vi "measure_max_power_stabilisation_keithley-2450.vi"(4 "Skip pixel?":bool, 5 "Date array":string[](array[string]), 6 "Scan settings":T1={"J-V scan"=TRUE, "Start voltage (V)"=0.0, "End voltage (V)"=0.0, "Step voltage (V)"=1.4, "Scan both directions"=TRUE, "Inverted device structure"=FALSE, "Settling delay (ms)"=10.0, "Measurement speed"=0, "Scan rate (V/s)"=0.0, "Stabilisation time (s)"=0.0, "Stabilisation mode"=0, "Stabilisation value (V or A) "=1.0, "Illumination"=0, "Stabilisation in the dark?"=FALSE, "Repeat light scans"=FALSE, "No. of repeat scans"=0.0, "Only repeat for best pixel"=1, "J-t scan"=FALSE, "J-t best pixel only"=7, "J-t start voltage (V)"=0.0, "J-t end voltage (V)"=1.4, "J-t step voltage (V)"=0.01, "Step time (s)"=0.7, "J-t scan both directions"=TRUE, "J-t inverted device structure"=FALSE, "J-t settling delay (ms)"=0.0, "J-t measurement speed"=0, "J-t illumination"=2, "Max. power stabilisation"=FALSE, "Max power best pixel only"=1, "Max. power point tracker"=FALSE, "Vmp from J-V scan"=FALSE, "Max P stab. Specific voltage"=FALSE, "Vmp (V)"=1.0, "Stabilisation time step (s)"=1.0, "Total stabilisation time (s)"=100.0} {"J-t settling delay (ms)" min=10.0; "J-t illumination" items=["Light only", "Dark only", "Light then dark", "Dark then light"]; "Measurement speed" items=["Fast", "Normal", "High accuracy"]; "Illumination" items=["Light only", "Dark only", "Light then dark", "Dark then light"]; "Only repeat for best pixel" items=["only for best pixel", "for best 2 pixels", "for best 3 pixels", "for best 4 pixels", "for best 5 pixels", "for best 6 pixels", "for best 7 pixels", "for all pixels"]; "No. of repeat scans" min=1.0 step=1.0; "Max power best pixel only" items=["only the best pixel", "the best 2 pixels", "the best 3 pixels", "the best 4 pixels", "the best 5 pixels", "the best 6 pixels", "the best 7 pixels", "all pixels"]; "J-t best pixel only" items=["only the best pixel", "the best 2 pixels", "the best 3 pixels", "the best 4 pixels", "the best 5 pixels", "the best 6 pixels", "the best 7 pixels", "all pixels"]; "J-t measurement speed" items=["Fast", "Normal", "High Accuracy"]; "Stabilisation mode" items=["V", "I"]; "Settling delay (ms)" min=10.0}, 7 "Cell details cluster":T2={"Cell Position"=16, "Cell Label"="", "Pixel to measure"=0, "Area (cm^2)"=0.126, "Variable"="", "Variable value"="", "Scan settings in queue"=0, "Light or dark"="", "Measurement Type"=""} {"Pixel to measure" items=["All", "1", "2", "3", "4", "5", "6", "7", "8"]}, 8 "Intensity (no. of suns)":string, 9 "File path of JV log":path, 10 "Experiment Title":string, 11 "User Name":string) -> (3 "Jt Curve":cluster{"Y":dbl[], "Y":dbl[]}[](graph) caption="JV Curve")   [LabVIEW 2016]
uses:
  TypeDefs/scan_settings.ctl
  <vilib>/Utility/file.llb/Read Delimited Spreadsheet (DBL).vi
  <instrlib>/Keithley 2450/Keithley 2450.lvlib
panel:
  out "File path for Jt image":path
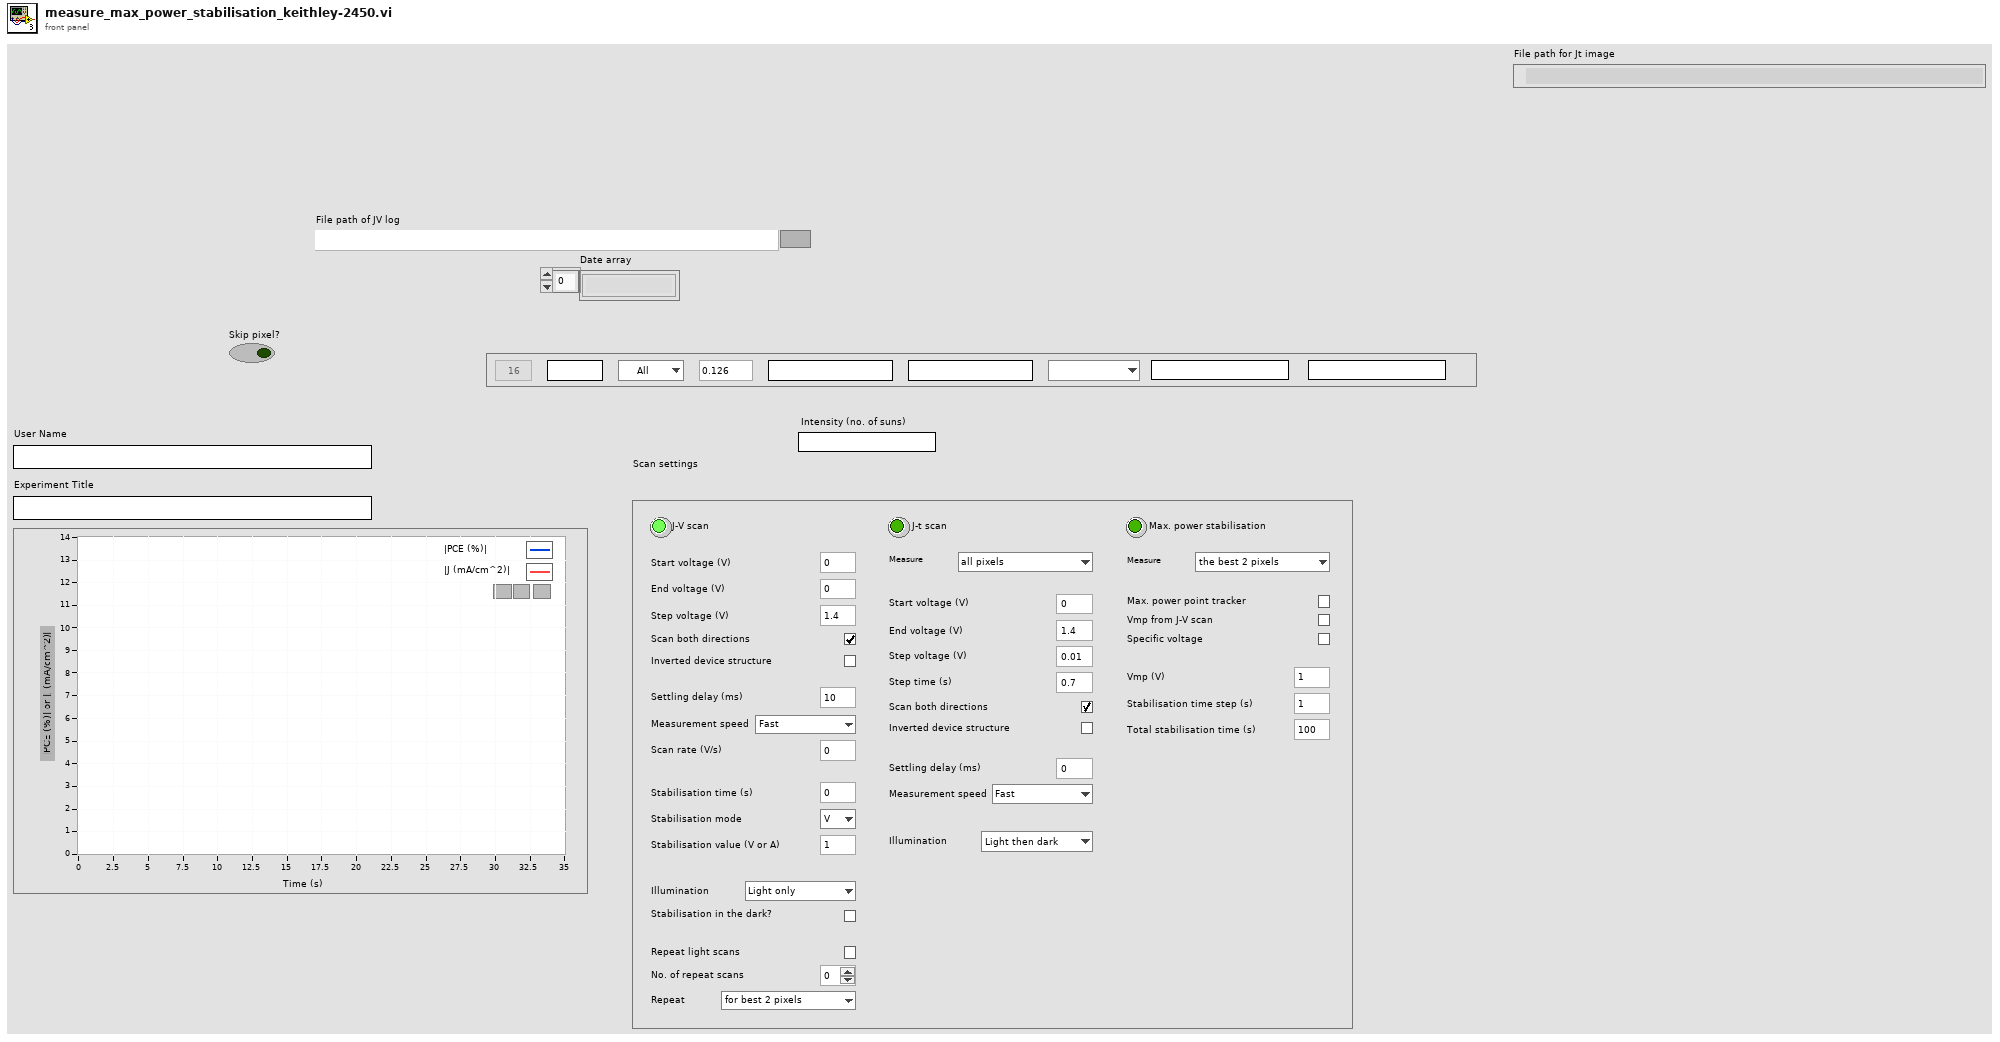
[diagram p1: front panel]
types:
  T1 = typedef "scan_settings.ctl" = cluster{"J-V scan":bool, "Start voltage (V)":dbl, "End voltage (V)":dbl, "Step voltage (V)":dbl, "Scan both directions":bool, "Inverted device structure":bool, "Settling delay (ms)":dbl, "Measurement speed":u8, "Scan rate (V/s)":dbl, "Stabilisation time (s)":dbl, "Stabilisation mode":u16, "Stabilisation value (V or A) ":dbl, "Illumination":u16, "Stabilisation in the dark?":bool, "Repeat light scans":bool, "No. of repeat scans":dbl, "Only repeat for best pixel":u16, "J-t scan":bool, "J-t best pixel only":u16, "J-t start voltage (V)":dbl, "J-t end voltage (V)":dbl, "J-t step voltage (V)":dbl, "Step time (s)":dbl, "J-t scan both directions":bool, "J-t inverted device structure":bool, "J-t settling delay (ms)":dbl, "J-t measurement speed":u16, "J-t illumination":u16, "Max. power stabilisation":bool, "Max power best pixel only":u16, "Max. power point tracker":bool, "Vmp from J-V scan":bool, "Max P stab. Specific voltage":bool, "Vmp (V)":dbl, "Stabilisation time step (s)":dbl, "Total stabilisation time (s)":dbl}
  T2 = cluster{"Cell Position":i32, "Cell Label":string, "Pixel to measure":u16, "Area (cm^2)":dbl, "Variable":string, "Variable value":string, "Scan settings in queue":u16, "Light or dark":string, "Measurement Type":string}
  T3 = typedef "imagedata.ctl" = cluster{"image type":i32, "image depth":i32, "image":u8[], "mask":u8[], "colors":u32[], "Rectangle":cluster{"left":i16, "top":i16, "right":i16, "bottom":i16}}
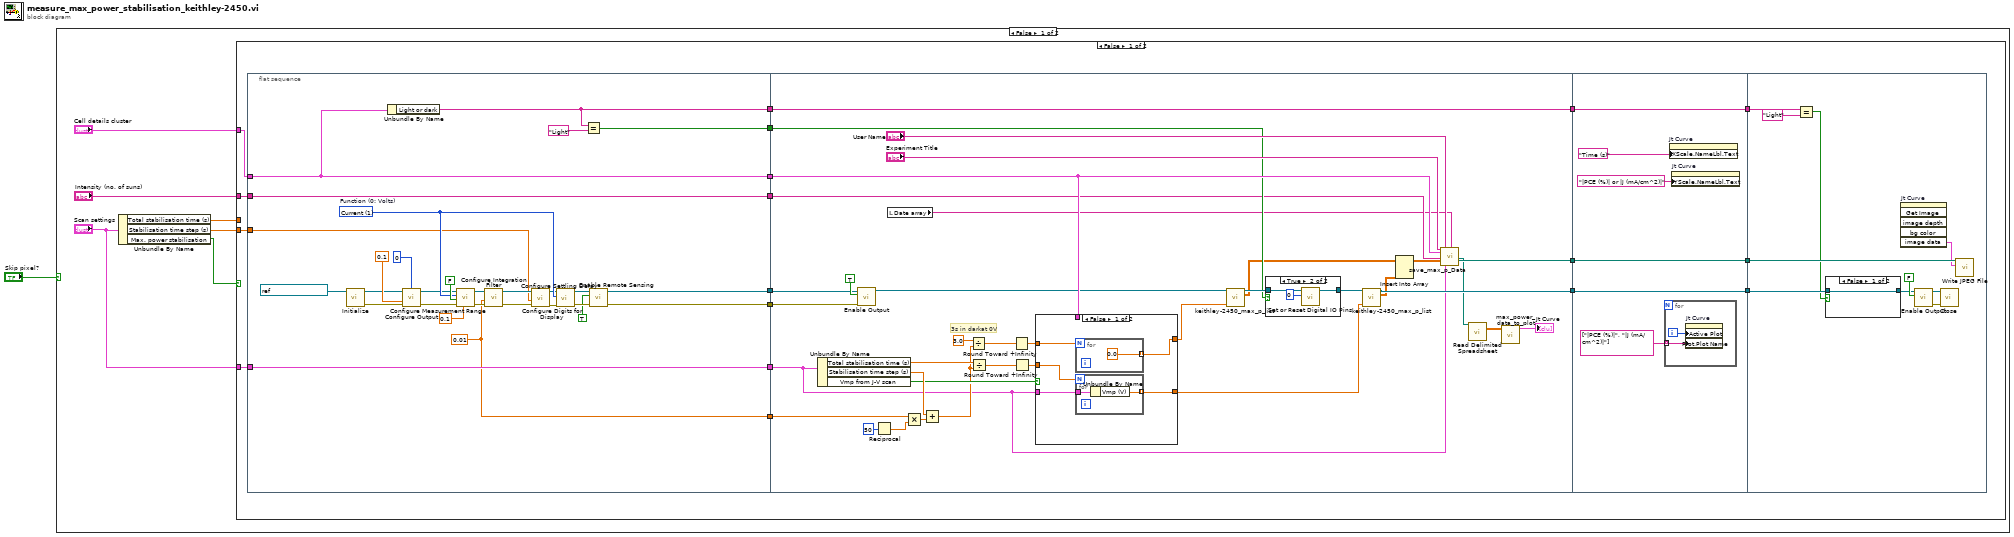
[diagram p0: block diagram]
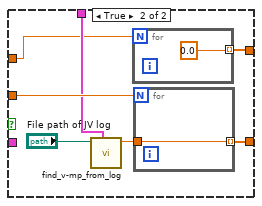
[diagram p3: hidden frame]
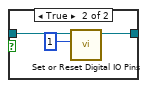
[diagram p4: hidden frame]
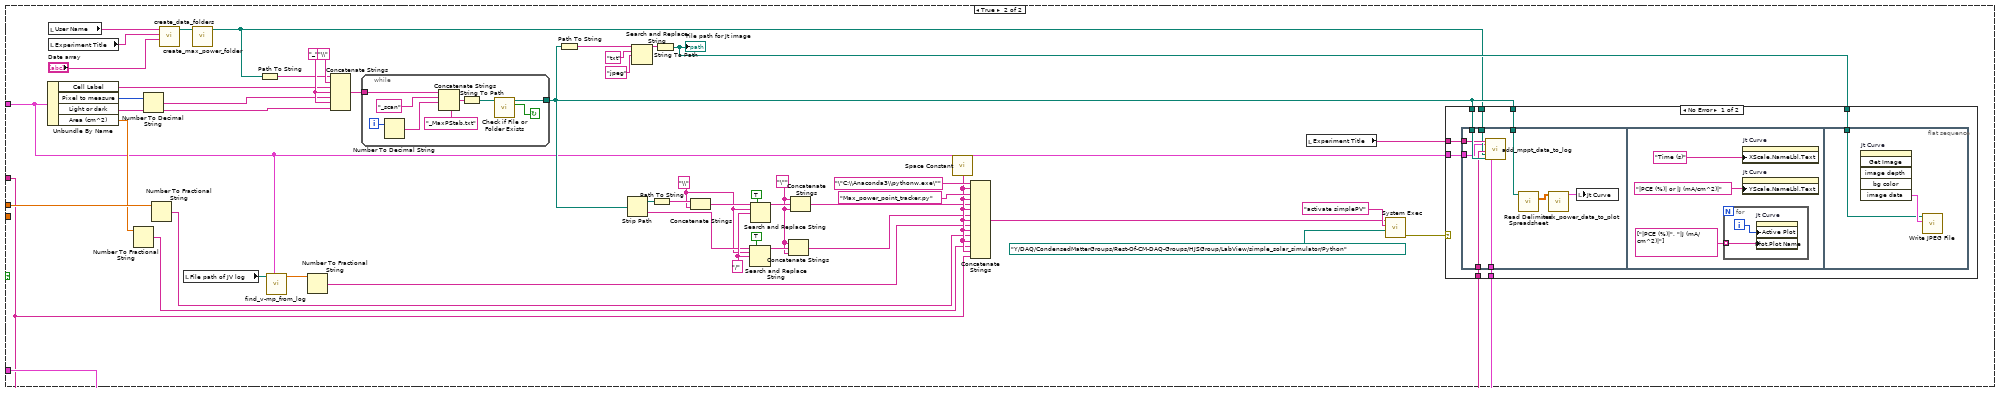
[diagram p5: hidden frame]
diagram:
  n1 = case shown="False" "Skip pixel?" {
    frame False {
      n2 = Unbundle By Name("Scan settings") -> ("Total stabilisation time (s)"=w3:dbl, "Stabilisation time step (s)"=w7:dbl, "Max. power stabilisation"=w4:bool)
      n3 = case shown="False" w4 {
        tunnel: w7 -> [w18 _]
        tunnel: "Cell details cluster" -> [w17 w148]
        tunnel: "Scan settings" -> [w16 w152]
        tunnel: w3 -> [_ w162]
        tunnel: "Intensity (no. of suns)" -> [w14 w136]
        frame False {
          n4 = flat-sequence {
            tunnel: [w26] -> w24
            tunnel: [w27] -> w25
            tunnel: [w37] -> w23
            tunnel: w18 -> [w38]
            tunnel: [w40] -> w22
            tunnel: w17 -> [w40]
            tunnel: [w42] -> w21
            tunnel: w16 -> [w42]
            tunnel: [w39] -> w20
            tunnel: [w36] -> w19
            tunnel: [w28] -> w15
            tunnel: w14 -> [w28]
            tunnel: [w89] -> w13
            tunnel: [w91] -> w11
            tunnel: w25 -> [w61]
            tunnel: w24 -> [w60]
            tunnel: w23 -> [w82]
            tunnel: w22 -> [w75]
            tunnel: w21 -> [w55]
            tunnel: [w85] -> w9
            tunnel: w20 -> [w85]
            tunnel: w19 -> [w65]
            tunnel: w15 -> [w59]
            tunnel: w13 -> [w118]
            tunnel: [w118] -> w12
            tunnel: w11 -> [w117]
            tunnel: [w117] -> w10
            tunnel: w9 -> [w116]
            tunnel: [w116] -> w8
            tunnel: w12 -> [w124]
            tunnel: w10 -> [w127]
            tunnel: w8 -> [w121]
            frame #0 {
              w34 = 0
              w37 = 0.01
              w47 = u16 1 items=["Volts", "Current", "Resistance"]  # Function (0: Volts)
              n5 = call <instrlib>:"Initialize.vi"("VISA resource name"=refnum<visa-resource-name> "GPIB1::24::INSTR") -> ("error out"=w29:errorcluster, "VISA resource name out"=w32:refnum<visa-resource-name>)  [unwired: 9 in]
              n6 = Unbundle By Name(w40) -> ("Light or dark"=w39:string)
              n7 = call <instrlib>:"Configure Output.vi"("VISA resource name"=w32, "Source Level (0)"=w34, "Source Mode  (0: Voltage)"=w34, "Source Limit Level (0.1)"=0.1, "error in (no error)"=w29) -> ("VISA resource name out"=w31:refnum<visa-resource-name>, "error out"=w30:errorcluster)  [unwired: 9 in]
              n8 = call <instrlib>:"Configure Measurement Range.vi"("Manual Range (1.0)"=0.1, "error in (no error)"=w30, "Enable Auto Range (T:Enable)"=FALSE, "Function (0: Volts)"=w47, "VISA resource name"=w31) -> ("error out"=w50:errorcluster, "VISA resource name out"=w49:refnum<visa-resource-name>)  [unwired: 5 in]
              n9 = call <instrlib>:"Configure Integration Filter.vi"("error in (no error)"=w50, "Measurement Speed (1 PLC)"=w37, "VISA resource name"=w49) -> ("error out"=w43:errorcluster, "VISA resource name out"=w46:refnum<visa-resource-name>)  [unwired: 7 in]
              n10 = call <instrlib>:"Configure Settling Delay.vi"("error in (no error)"=w43, "Manual Delay (0 sec)"=w38, "VISA resource name"=w46) -> ("error out"=w44:errorcluster, "VISA resource name out"=w45:refnum<visa-resource-name>)  [unwired: 7 in]
              n11 = call <instrlib>:"Configure Digits for Display.vi"("error in (no error)"=w44, "Function (0: Volts)"=w47, "VISA resource name"=w45) -> ("error out"=w52:errorcluster, "VISA resource name out"=w51:refnum<visa-resource-name>)  [unwired: 7 in]
              n12 = Equal?(x=w39, y="Light") -> (x = y?=w36:bool)
              n13 = call <instrlib>:"Enable Remote Sensing.vi"("error in (no error)"=w52, "Enable Remote Sensing (T: Enable)"=TRUE ("Enable Output (T: Enable)"), "VISA resource name"=w51) -> ("error out"=w26:errorcluster, "VISA resource name out"=w27:refnum<visa-resource-name>)  [unwired: 7 in]
            }
            frame #1 {
              # "3s in darkat 0V"
              n14 = Unbundle By Name(w55) -> ("Total stabilisation time (s)"=w79:dbl, "Stabilisation time step (s)"=w80:dbl, "Vmp from J-V scan"=w76:bool)
              n15 = call <instrlib>:"Enable Output.vi"("error in (no error)"=w60, "Enable Output (T: Enable)"=TRUE ("Output (Off)"), "VISA resource name"=w61) -> ("VISA resource name out"=w67:refnum<visa-resource-name>)  [unwired: 7 in, 1 out]
              n16 = Reciprocal(x=50) -> (1/x=w84:dbl)
              n17 = local read "Date array"() -> (w56:string[])
              n18 = Multiply(x=w82, y=w84) -> (x*y=w81:dbl)
              n19 = Add(x=w80, y=w81) -> (x+y=w74:dbl)
              n20 = Divide(x=3.0, y=w74) -> (x/y=w71:dbl)
              n21 = Divide(x=w79, y=w74) -> (x/y=w72:dbl)
              n22 = Round Toward +Infinity(x=w71) -> (ceil(x): smallest int >= x=w70:dbl)
              n23 = Round Toward +Infinity(x=w72) -> (ceil(x): smallest int >= x=w78:dbl)
              n24 = case shown="False" w76 {
                tunnel: w78 -> [w100 w109]
                tunnel: w55 -> [w98 _]
                tunnel: [w99 w108] -> w77
                tunnel: w75 -> [_ w107]
                tunnel: w70 -> [w97 w106]
                tunnel: [w96 w105] -> w68
                frame False {
                  n25 = for {
                    N: w97 -> [_]
                    tunnel: [0.0 ("Vmp")] -> w96 mode=indexing
                  }
                  n26 = for {
                    N: w100 -> [_]
                    tunnel: w98 -> [w103]
                    tunnel: [w102] -> w99 mode=indexing
                    n27 = Unbundle By Name(w103) -> ("Vmp (V)"=w102:dbl)
                  }
                }
                frame True {
                  n28 = call "find_v-mp_from_log.vi"("Cell details cluster in"=w107, "File path of JV log"="File path of JV log") -> ("Vmp"=w104:dbl)  [unwired: 9 in]
                  n29 = for {
                    N: w106 -> [_]
                    tunnel: [0.0 ("Vmp")] -> w105 mode=indexing
                  }
                  n30 = for {
                    N: w109 -> [_]
                    tunnel: [w112] -> w108 mode=indexing
                    tunnel: w104 -> [w112]
                  }
                }
              }
              n31 = call "keithley-2450_max_p_list.vi"("VISA resource name in"=w67, "Voltage List"=w68) -> ("VISA resource name out"=w66:refnum<visa-resource-name>, "Data Array"=w64:dbl[][])  [unwired: 11 in, 1 out]
              n32 = case shown="True" w65 {
                tunnel: w66 -> [w92 w94]
                tunnel: [w92 w93] -> w69
                frame False {
                }
                frame True {
                  n33 = call <instrlib>:"Set or Reset Digital IO Pins.vi"("Digital IO Line (1)"=0, "VISA resource name"=w94) -> ("VISA resource name out"=w93:refnum<visa-resource-name>)  [unwired: 8 in, 1 out]
                }
              }
              n34 = call "keithley-2450_max_p_list.vi"("VISA resource name in"=w69, "Voltage List"=w77) -> ("VISA resource name out"=w89:refnum<visa-resource-name>, "Data Array"=w63:dbl[][])  [unwired: 11 in, 1 out]
              n35 = Insert Into Array(array=w64, new element=w63) -> (w62:dbl[][])  [unwired: 2 in]
              n36 = call "save_max_p_Data.vi"("Experiment Indicator"="Experiment Title", "Cell details cluster"=w75, "Intensity (no. of suns)"=w59, "Data Array"=w62, "Username"="User Name", "Scan settings"=w55, "Date array"=w56) -> ("File path for Jt data"=w58:path, "File path for Jt image"=w91:path)  [unwired: 9 in, 2 out]
              n37 = call-poly <vilib>:"Read Delimited Spreadsheet.vi"("file path (dialog if empty)"=w58) -> ("all rows"=w57:dbl[][])  [unwired: 9 in, 5 out]
              n38 = call "max_power_data_to_plot.vi"("Data Array"=w57) -> ("JV Curve"=→"Jt Curve":cluster{"Y":dbl[], "Y":dbl[]}[])  [unwired: 10 in]
            }
            frame #2 {
              n39 = for {
                tunnel: string[] ["|PCE (%)|", "|J (mA/cm^2)|"] ("Measurement queue") -> [w119] mode=indexing
                i -> [w120]
                n40 = property on="Jt Curve" class="XYGraph (strict)"("Active Plot"=w120, "Plot.Plot Name"=w119) -> ()  [unwired: 2 in, 2 out]
              }
              n41 = property on="Jt Curve" class="XYGraph (strict)"("XScale.NameLbl.Text"="Time (s)" ("Y Scale.Name Label.Text")) -> ()  [unwired: 2 in, 2 out]
              n42 = property on="Jt Curve" class="XYGraph (strict)"("YScale.NameLbl.Text"="|PCE (%)| or |J (mA/cm^2)|" ("Y Scale.Name Label.Text")) -> ()  [unwired: 2 in, 2 out]
            }
            frame #3 {
              n43 = Equal?(x=w121, y="Light") -> (x = y?=w122:bool)
              n44 = case shown="False" w122 {
                tunnel: w124 -> [w131 w133]
                tunnel: [w131 w132] -> w123
                frame False {
                }
                frame True {
                  n45 = call <instrlib>:"Set or Reset Digital IO Pins.vi"("Digital IO Line (1)"=1, "VISA resource name"=w133) -> ("VISA resource name out"=w132:refnum<visa-resource-name>)  [unwired: 8 in, 1 out]
                }
              }
              n46 = invoke on="Jt Curve" class="XYGraph (strict)" method="Get Image"() -> ("image data"=w126:T3)  [unwired: 6 in, 5 out]
              n47 = call <instrlib>:"Enable Output.vi"("Enable Output (T: Enable)"=FALSE ("Output (Off)"), "VISA resource name"=w123) -> ("error out"=w129:errorcluster, "VISA resource name out"=w130:refnum<visa-resource-name>)  [unwired: 8 in]
              n48 = call <instrlib>:"Close.vi"("error in (no error)"=w129, "VISA resource name"=w130) -> ()  [unwired: 9 in, 1 out]
              n49 = call <vilib>:"Write JPEG File.vi"("image data"=w126, "path to JPEG file"=w127) -> ()  [unwired: 8 in, 2 out]
            }
          }
        }
        frame True {
          w143 = "\"" ("string")
          w167 = "/" ("search string")
          w142 = "\\" ("search string")
          w177 = "_"
          n50 = Unbundle By Name(w148) -> ("Cell Label"=w173:string, "Pixel to measure"=w174:u16, "Light or dark"=w171:string, "Area (cm^2)"=w159:dbl)
          n51 = local read "User Name"() -> (w179:string)
          n52 = local read "Experiment Title"() -> (w180:string)
          n53 = Number To Fractional String(number=w159) -> (F-format string=w137:string)  [unwired: 3 in]
          n54 = Number To Decimal String(number=w174) -> (decimal integer string=w172:string)  [unwired: 1 in]
          n55 = Number To Fractional String(number=w162) -> (F-format string=w138:string)  [unwired: 3 in]
          n56 = call "create_data_folders.vi"("Date array"="Date array", "Experiment Indicator"=w180, "username"=w179) -> ("Data Output Folder"=w178:path)  [unwired: 8 in]
          n57 = local read "File path of JV log"() -> (w161:path)
          n58 = call "create_max_power_folder.vi"("Data Folder In"=w178) -> ("Data Output Folder"=w149:path)  [unwired: 10 in]
          n59 = Path To String(path=w149) -> (string=w168:string)
          n60 = call "find_v-mp_from_log.vi"("Cell details cluster in"=w148, "File path of JV log"=w161) -> ("Vmp"=w160:dbl)  [unwired: 9 in]
          n61 = Number To Fractional String(number=w160) -> (F-format string=w139:string)  [unwired: 3 in]
          n62 = Concatenate Strings(w168, "\\", w173, w177, w172, w177, w171) -> (w176:string)
          n63 = while {
            tunnel: w176 -> [w217]
            tunnel: [w209] -> w151
            i -> [w215]
            stop <- w210 continue-if-true
            n64 = Number To Decimal String(number=w215) -> (decimal integer string=w214:string)  [unwired: 1 in]
            n65 = Concatenate Strings(w217, "_scan", w214, "_MaxPStab.txt") -> (w211:string)
            n66 = String To Path(string=w211) -> (path=w212:path)
            n67 = call <vilib>:"Check if File or Folder Exists.vi"("path"=w212) -> ("file or folder exists?"=w210:bool, "dup path"=w209:path)  [unwired: 8 in, 1 out]
          }
          n68 = Path To String(path=w151) -> (string=w184:string)
          n69 = Strip Path(path=w151) -> (stripped path=w157:path, name=w158:string)
          n70 = Search and Replace String(input string=w184, search string="txt", replace string="jpeg") -> (result string=w181:string)  [unwired: 5 in, 3 out]
          n71 = Path To String(path=w157) -> (string=w155:string)
          n72 = String To Path(string=w181) -> (path=w163:path)
          "File path for Jt image" <- w163
          n73 = Concatenate Strings(w155, w142) -> (w156:string)
          n74 = Search and Replace String(replace all?=TRUE ("replace all? (F)"), input string=w158, search string=w142, replace string=w167) -> (result string=w165:string)  [unwired: 4 in, 3 out]
          n75 = Search and Replace String(replace all?=TRUE ("replace all? (F)"), input string=w156, search string=w142, replace string=w167) -> (result string=w170:string)  [unwired: 4 in, 3 out]
          n76 = Concatenate Strings(w143, w165, w143) -> (w140:string)
          n77 = Concatenate Strings(w143, w170, w143) -> (w141:string)
          n78 = call <vilib>:"Space Constant.vi"() -> ("String"=w144:string)
          n79 = Concatenate Strings("\"C:\\Anaconda3\\pythonw.exe\"" ("standard input"), w144, "Max_power_point_tracker.py" ("standard input"), w144, w141, w144, w140, w144, w139, w144, w138, w144, w137, w144, w136) -> (w135:string)
          n80 = local read "Experiment Title"() -> (w150:string)
          n81 = call <vilib>:"System Exec.vi"("working directory"=path "Y:/DAQ/CondensedMatterGroups/Rest-Of-CM-DAQ-Groups/HJSGroup/LabView/simple_solar_simulator/Python", "standard input"="activate simplePV", "command line"=w135) -> ("error out"=w164:errorcluster)  [unwired: 5 in, 3 out]
          n82 = case shown="No Error" w164 {
            tunnel: w151 -> [w192 _]
            tunnel: w163 -> [w191 _]
            tunnel: w152 -> [w190 _]
            tunnel: w151 -> [w189 _]
            tunnel: w136 -> [w188 _]
            tunnel: w150 -> [w187 _]
            tunnel: w149 -> [w186 _]
            tunnel: w148 -> [w185 _]
            frame No Error {
              n83 = flat-sequence {
                tunnel: w192 -> [w201]
                tunnel: w190 -> [w198]
                tunnel: w189 -> [w197]
                tunnel: w188 -> [w196]
                tunnel: w187 -> [w195]
                tunnel: w186 -> [w194]
                tunnel: w185 -> [w193]
                tunnel: w191 -> [w207]
                frame #0 {
                  n84 = call "add_mppt_data_to_log.vi"("Experiment Indicator"=w195, "Cell details cluster"=w193, "Intensity (no. of suns)"=w196, "mppt folder path"=w194, "mppt file path"=w197, "Scan settings"=w198) -> ()  [unwired: 12 in, 2 out]
                  n85 = call-poly <vilib>:"Read Delimited Spreadsheet.vi"("file path (dialog if empty)"=w201) -> ("all rows"=w200:dbl[][])  [unwired: 9 in, 5 out]
                  n86 = call "max_power_data_to_plot.vi"("Data Array"=w200) -> ("JV Curve"=w199:cluster{"Y":dbl[], "Y":dbl[]}[])  [unwired: 10 in]
                  n87 = local write "Jt Curve"(w199) -> ()
                }
                frame #1 {
                  n88 = for {
                    tunnel: string[] ["|PCE (%)|", "|J (mA/cm^2)|"] ("Measurement queue") -> [w205] mode=indexing
                    i -> [w206]
                    n89 = property on="Jt Curve" class="XYGraph (strict)"("Active Plot"=w206, "Plot.Plot Name"=w205) -> ()  [unwired: 2 in, 2 out]
                  }
                  n90 = property on="Jt Curve" class="XYGraph (strict)"("XScale.NameLbl.Text"="Time (s)" ("Y Scale.Name Label.Text")) -> ()  [unwired: 2 in, 2 out]
                  n91 = property on="Jt Curve" class="XYGraph (strict)"("YScale.NameLbl.Text"="|PCE (%)| or |J (mA/cm^2)|" ("Y Scale.Name Label.Text")) -> ()  [unwired: 2 in, 2 out]
                }
                frame #2 {
                  n92 = invoke on="Jt Curve" class="XYGraph (strict)" method="Get Image"() -> ("image data"=w208:T3)  [unwired: 6 in, 5 out]
                  n93 = call <vilib>:"Write JPEG File.vi"("image data"=w208, "path to JPEG file"=w207) -> ()  [unwired: 8 in, 2 out]
                }
              }
            }
            frame Error {
            }
          }
        }
      }
    }
    frame True {
    }
  }
